vi "BlinkM ReadScriptLine.vi"(0 "Arduino Resource":T1={"VISA resource"="", "Board Type"=enum."Uno", "Connection Type"=enum."USB / Serial", "Bytes Per Packet (15)"=15}, 5 "Address":u8, 7 "BlinkM Script (User Script)":T4, 9 "Script Line (0)":u8, 11 "error in":errorcluster) -> (4 "Arduino Resource":T1={"VISA resource"="", "Board Type"=enum."Uno", "Connection Type"=enum."USB / Serial", "Bytes Per Packet (15)"=15}, 8 "BlinkM Script Line":T3, 15 "error out":errorcluster)   [LabVIEW 2015, in "LabVIEW Interface for Arduino.lvlib"]
doc: "Read a light script line from the specified BlinkM, lightscript and line.s"
uses:
  <vilib>/LabVIEW Interface for Arduino/LabVIEW Interface for Arduino.lvlib
  <vilib>/LabVIEW Interface for Arduino/Type Defs/BlinkM Script.ctl
  <vilib>/LabVIEW Interface for Arduino/Type Defs/Arduino Resource.ctl
  <vilib>/LabVIEW Interface for Arduino/Type Defs/Board Type.ctl
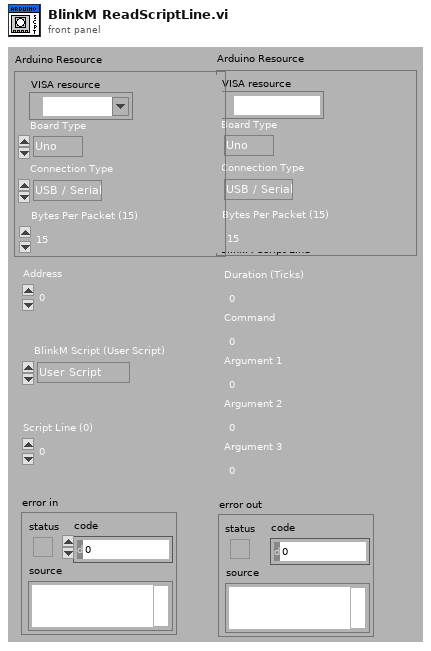
[diagram p1: front panel]
types:
  T1 = typedef "LabVIEW Interface for Arduino.lvlib/Arduino Resource.ctl" = cluster{"VISA resource":refnum<visa-resource-name>, "Board Type":T2, "Connection Type":enum8{"USB / Serial"}, "Bytes Per Packet (15)":u8}
  T2 = typedef "LabVIEW Interface for Arduino.lvlib/Board Type.ctl" = enum16{"Uno", "Dimuelanove w/Atmega 328", "Mega 2560"}
  T3 = cluster{"Duration (Ticks)":u8, "Command":u8, "Argument 1":u8, "Argument 2":u8, "Argument 3":u8}
  T4 = typedef "LabVIEW Interface for Arduino.lvlib/BlinkM Script.ctl" = enum8{"User Script", "RGB", "White Flash", "Red Flash", "Green Flash", "Blue Flash", "Cyan Flash", "Magenta Flash", "Yellow Flash", "Black", "Hue Cycle", "Mood Light", "Virtual Candle", "Water Reflections", "Old Neon", "The Seasons", "Thunderstorm", "Stop Light", "Morse Code S.O.S"}
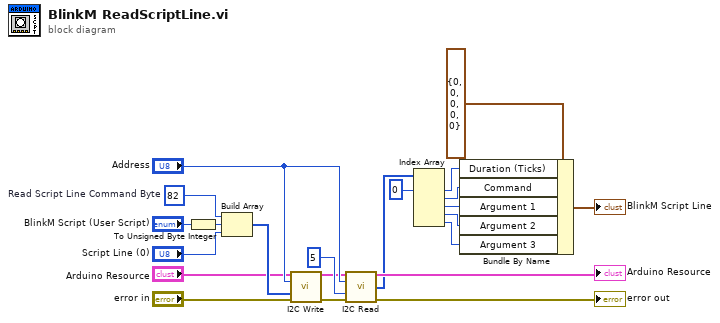
[diagram p0: block diagram]
diagram:
  w21 = u8 82  # Read Script Line Command Byte
  n1 = To Unsigned Byte Integer(number="BlinkM Script (User Script)") -> (unsigned 8bit integer=w7:u8)
  n2 = Build Array(w21, w7, "Script Line (0)") -> (w20:u8[])
  n3 = call <vilib>:"I2C Write.vi"("Arduino Resource"="Arduino Resource", "Address (0)"="Address", "I2C Data Bytes"=w20, "error in"="error in") -> ("Arduino Resource"=w3:T1, "error out"=w18:errorcluster)  [unwired: 10 in]
  n4 = call <vilib>:"I2C Read.vi"("Arduino Resource"=w3, "Address (0)"="Address", "Bytes To Read"=u8 5, "error in"=w18) -> ("Arduino Resource"=→"Arduino Resource":T1, "I2C Data"=w1:u8[], "error out"=→"error out":errorcluster)  [unwired: 9 in]
  n5 = Index Array(array=w1, index #1=0 ("index")) -> (element #1=w13:u8, element #2=w12:u8, element #3=w11:u8, element #4=w10:u8, element #5=w9:u8)  [unwired: 4 in]
  n6 = Bundle By Name(cluster=T3 {"Duration (Ticks)"=0, "Command"=0, "Argument 1"=0, "Argument 2"=0, "Argument 3"=0}, "Duration (Ticks)"=w13, "Command"=w12, "Argument 1"=w11, "Argument 2"=w10, "Argument 3"=w9) -> (→"BlinkM Script Line":T3)
